vi "System7PressureTemp.vi"() -> ()   [LabVIEW 2015]
uses:
  Control 1.ctl
  <vilib>/DAQmx/write.llb/DAQmx Write (Digital 1D Bool NChan 1Samp 1Line).vi
  <vilib>/DAQmx/write.llb/DAQmx Write (Digital Bool 1Line 1Point).vi
  <vilib>/DAQmx/read.llb/DAQmx Read (Analog DBL 1Chan 1Samp).vi
  <vilib>/DAQmx/read.llb/DAQmx Read (Analog 1D Wfm NChan NSamp).vi
  <vilib>/Analysis/baseanly.llb/Mean (DBL).vi
  <vilib>/DAQmx/write.llb/DAQmx Write (Analog DBL 1Chan 1Samp).vi
  <vilib>/DAQmx/miscellaneous.llb/DAQmx Fill In Error Info.vi
  <vilib>/addons/control/pid/NI_PID_autopid.lvlib
  <vilib>/Analysis/NI_AALBase.lvlib
panel:
  out "Voltage Reading(Temp) 2":dbl format="%#_13g"
  out "Temperature (Celcius) 2":dbl format="%#.1g"
  out "Temp(C) 2":dbl(slide) scale=-10.0..100.0
  out "Temp Chart 3":waveform(dbl)(graph)
  in  "autotuning parameters 4":T1={"controller type"=1, "relay cycles"=3, "relay amplitude"=1.0, "control specification"=2, "PV noise level"=0.1} {"PV noise level" format="%.2f"; "control specification" items=["normal", "fast", "slow"]; "relay amplitude" format="%.2f"; "controller type" items=["PID", "PI", "P"]}
  in  "PID gains 4":T2={"proportional gain (Kc)"=1.0, "integral time (Ti, min)"=0.01, "derivative time (Td, min)"=0.0} {"derivative time (Td, min)" format="%.3f"; "integral time (Ti, min)" format="%.3f"; "proportional gain (Kc)" format="%.3f"}
  out "PID gains out 4":T2={"proportional gain (Kc)"=1.0, "integral time (Ti, min)"=0.01, "derivative time (Td, min)"=0.0} {"derivative time (Td, min)" format="%.3f"; "integral time (Ti, min)" format="%.3f"; "proportional gain (Kc)" format="%.3f"}
  in  "autotune? (F) 4":bool
  in  "reinitialize? (F) 4":bool
  in  "setpoint in C 2":dbl format="%.2f"
  in  "Manual Control 4":bool
  in  "Heater On/Off 2":bool
  out "Voltage Reading(Temp)":dbl format="%#_13g"
  out "Temperature (Celcius)":dbl format="%#.1g"
  out "Temp(C)":dbl(slide) scale=-10.0..100.0
  out "Temp Chart 2":waveform(dbl)(graph)
  in  "autotuning parameters 3":T1={"controller type"=1, "relay cycles"=3, "relay amplitude"=1.0, "control specification"=2, "PV noise level"=0.1} {"PV noise level" format="%.2f"; "control specification" items=["normal", "fast", "slow"]; "relay amplitude" format="%.2f"; "controller type" items=["PID", "PI", "P"]}
  in  "PID gains 3":T2={"proportional gain (Kc)"=1.0, "integral time (Ti, min)"=0.01, "derivative time (Td, min)"=0.0} {"derivative time (Td, min)" format="%.3f"; "integral time (Ti, min)" format="%.3f"; "proportional gain (Kc)" format="%.3f"}
  out "PID gains out 3":T2={"proportional gain (Kc)"=1.0, "integral time (Ti, min)"=0.01, "derivative time (Td, min)"=0.0} {"derivative time (Td, min)" format="%.3f"; "integral time (Ti, min)" format="%.3f"; "proportional gain (Kc)" format="%.3f"}
  in  "autotune? (F) 3":bool
  in  "reinitialize? (F) 3":bool
  in  "setpoint in C":dbl format="%.2f"
  out "Control Value 3":dbl
  in  "Manual Control 3":bool
  in  "Heater On/Off":bool
  in  "Open/Close (Green)":bool
  in  "Open/Close (Blue)":bool
  in  "Stop program":bool
  in  "On/Off":bool
  in  "Manual Control 2":bool
  in  "Voltage setting 2":dbl format="%#_13g"
  out "Voltage Reading(pressure) 2":dbl format="%#_13g"
  out "Pressure 2":dbl format="%#.3g"
  out "Pressure Chart 2":dbl(graph)
  in  "autotuning parameters 2":T1={"controller type"=1, "relay cycles"=3, "relay amplitude"=1.0, "control specification"=2, "PV noise level"=0.1} {"PV noise level" format="%.2f"; "control specification" items=["normal", "fast", "slow"]; "relay amplitude" format="%.2f"; "controller type" items=["PID", "PI", "P"]}
  in  "PID gains 2":T2={"proportional gain (Kc)"=1.0, "integral time (Ti, min)"=0.01, "derivative time (Td, min)"=0.0} {"derivative time (Td, min)" format="%.3f"; "integral time (Ti, min)" format="%.3f"; "proportional gain (Kc)" format="%.3f"}
  out "PID gains out 2":T2={"proportional gain (Kc)"=1.0, "integral time (Ti, min)"=0.01, "derivative time (Td, min)"=0.0} {"derivative time (Td, min)" format="%.3f"; "integral time (Ti, min)" format="%.3f"; "proportional gain (Kc)" format="%.3f"}
  in  "autotune? (F) 2":bool
  in  "reinitialize? (F) 2":bool
  in  "setpoint in Bar 2":dbl format="%#.5f"
  out "Control Value 2":dbl
  in  "Voltage setting":dbl format="%#_13g"
  in  "Manual Control":bool
  out "Control Value":dbl
  in  "setpoint in Bar":dbl format="%#.5f"
  in  "reinitialize? (F)":bool
  in  "autotune? (F)":bool
  out "PID gains out":T2={"proportional gain (Kc)"=1.0, "integral time (Ti, min)"=0.01, "derivative time (Td, min)"=0.0} {"derivative time (Td, min)" format="%.3f"; "integral time (Ti, min)" format="%.3f"; "proportional gain (Kc)" format="%.3f"}
  in  "PID gains":T2={"proportional gain (Kc)"=1.0, "integral time (Ti, min)"=0.01, "derivative time (Td, min)"=0.0} {"derivative time (Td, min)" format="%.3f"; "integral time (Ti, min)" format="%.3f"; "proportional gain (Kc)" format="%.3f"}
  in  "autotuning parameters":T1={"controller type"=1, "relay cycles"=3, "relay amplitude"=1.0, "control specification"=2, "PV noise level"=0.1} {"PV noise level" format="%.2f"; "control specification" items=["normal", "fast", "slow"]; "relay amplitude" format="%.2f"; "controller type" items=["PID", "PI", "P"]}
  out "Pressure Chart":dbl(graph)
  out "Pressure":dbl format="%#.3g"
  out "Voltage Reading(pressure)":dbl format="%#_13g"
  # "Valves"
  # "Pump 3"
  # "Pressure Vessel 2"
  # "Pressure Vessel 1"
  # "Readings"
  # "Controls"
  # "Readings"
  # "Controls"
  # "PID Settings"
  # "51.12139\n\n0.044676"
  # "Temperature 1"
  # "Temperature 2"
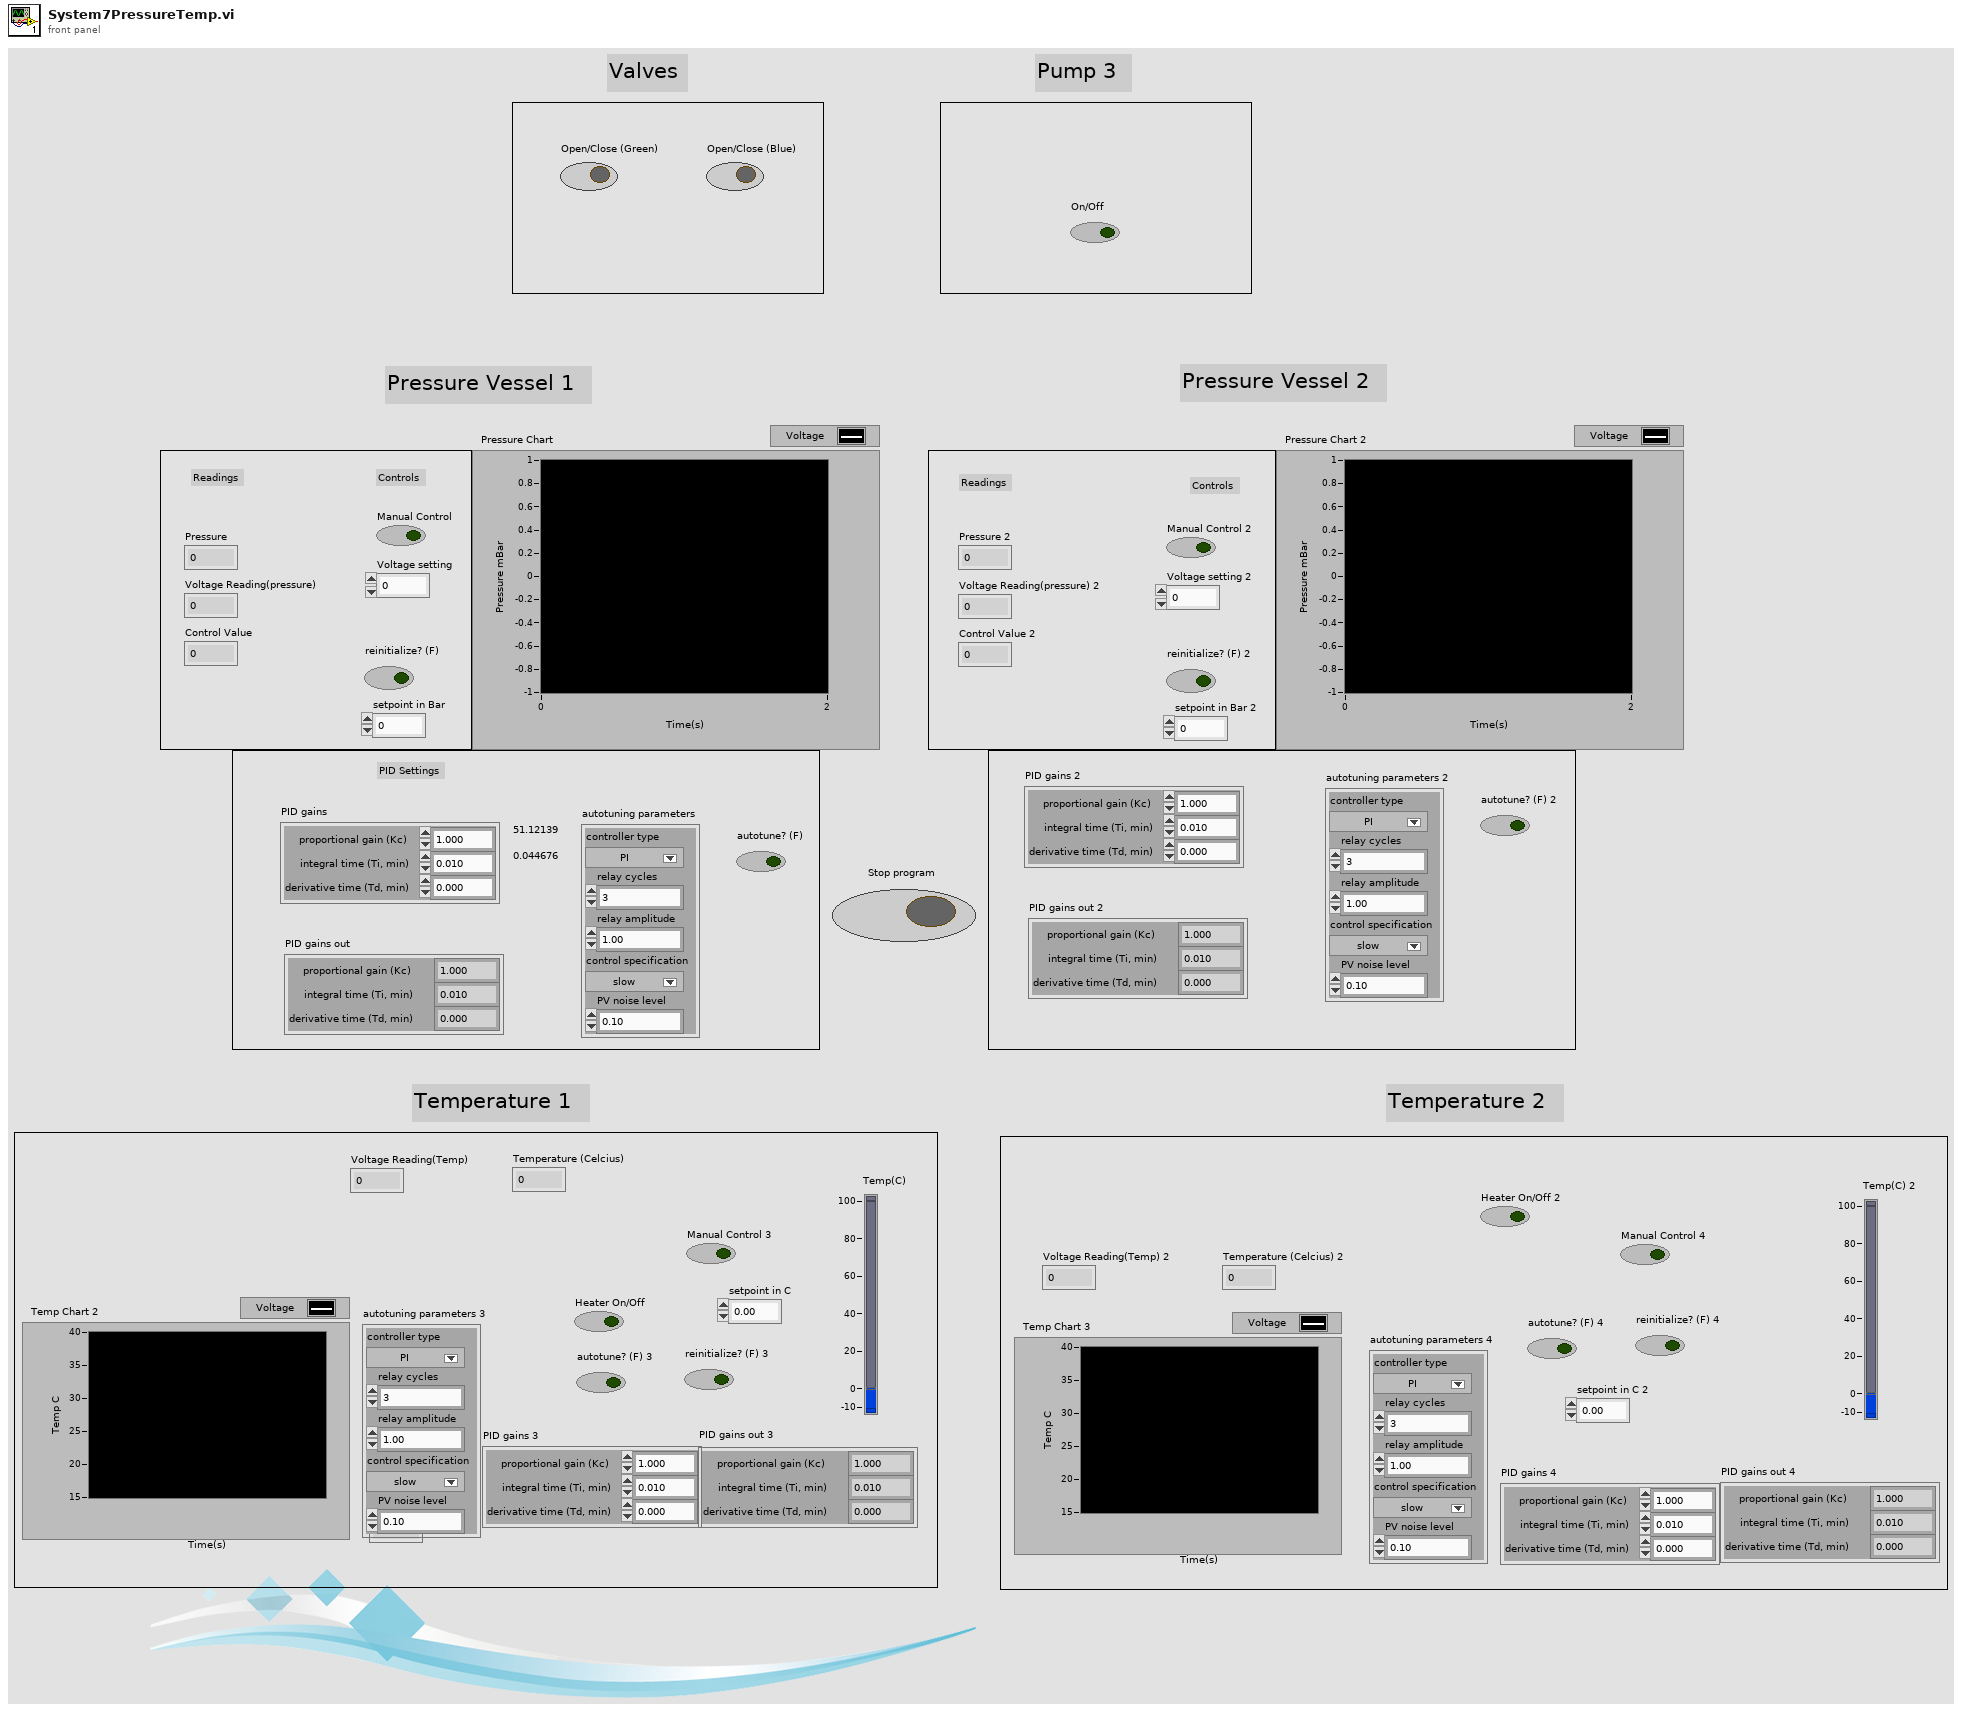
[diagram p1: front panel]
types:
  T1 = cluster{"controller type":u16, "relay cycles":i32, "relay amplitude":dbl, "control specification":u16, "PV noise level":dbl}
  T2 = cluster{"proportional gain (Kc)":dbl, "integral time (Ti, min)":dbl, "derivative time (Td, min)":dbl}
  T3 = typedef "Control 1.ctl" = refnum<k21>
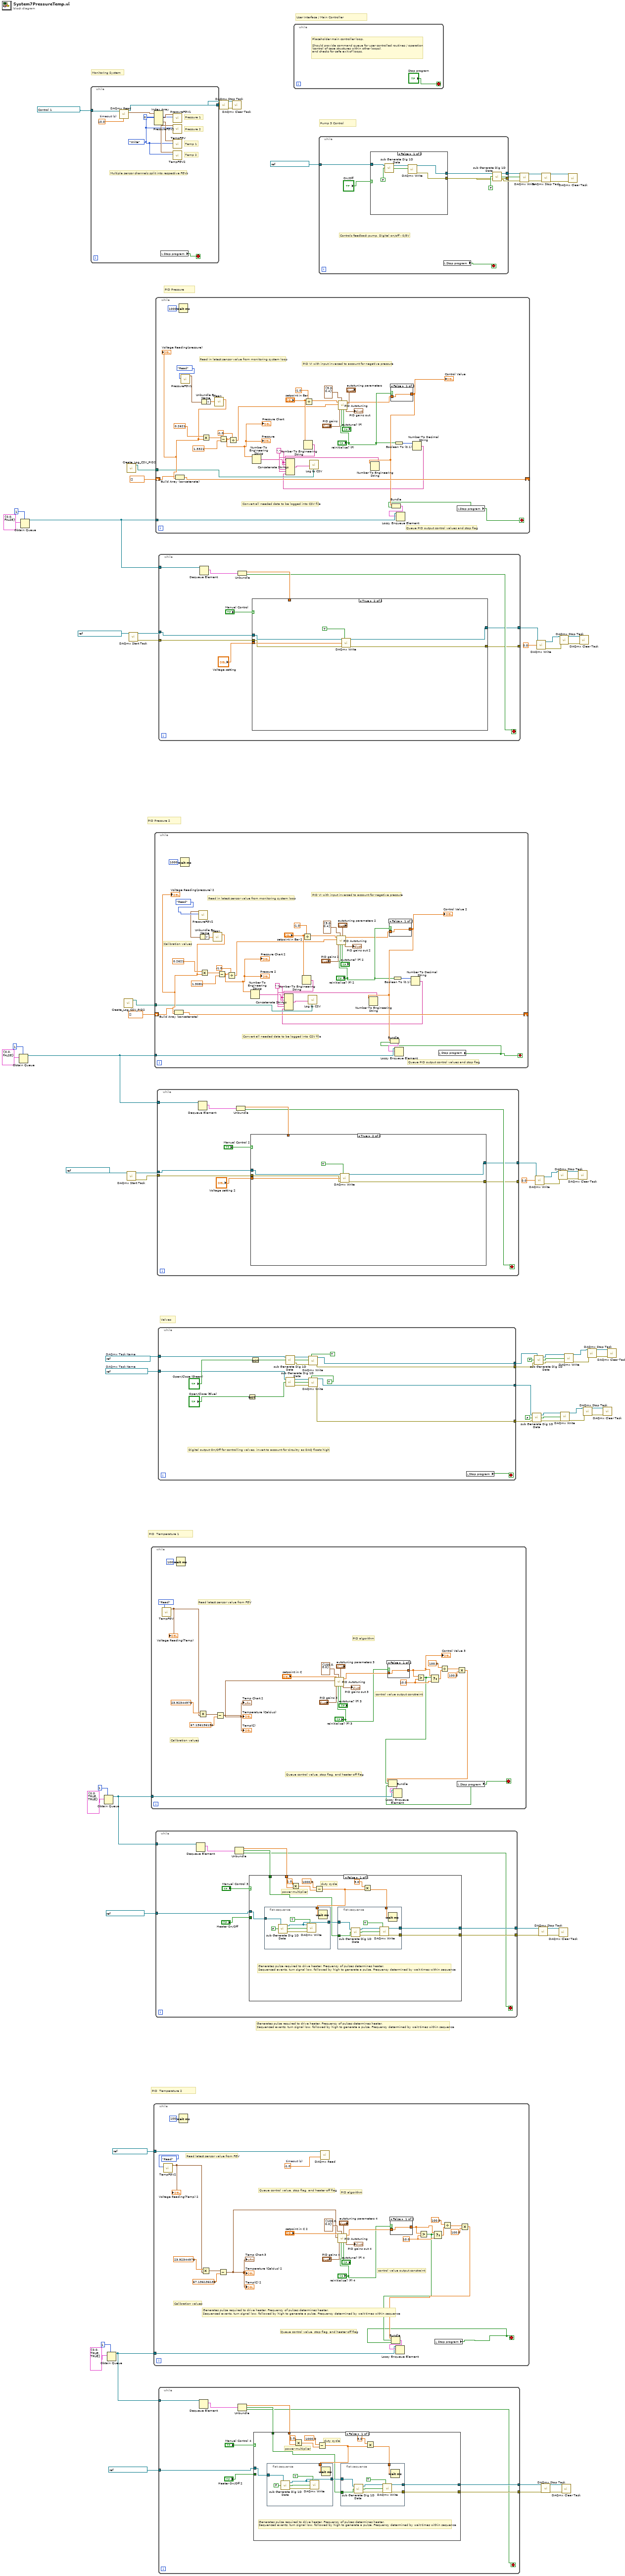
[diagram p0: block diagram]
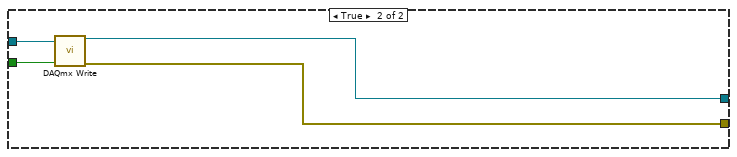
[diagram p2: hidden frame]
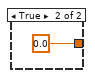
[diagram p3: hidden frame]
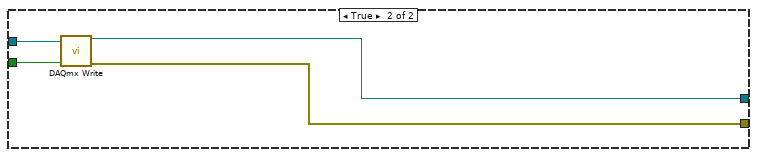
[diagram p4: hidden frame]
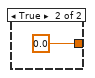
[diagram p5: hidden frame]
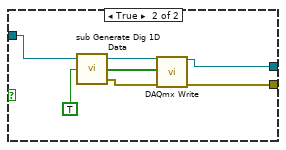
[diagram p6: hidden frame]
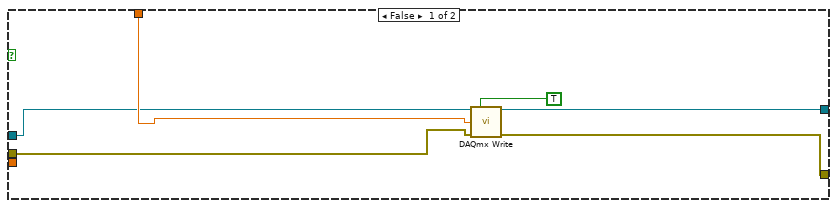
[diagram p7: hidden frame]
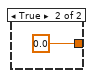
[diagram p8: hidden frame]
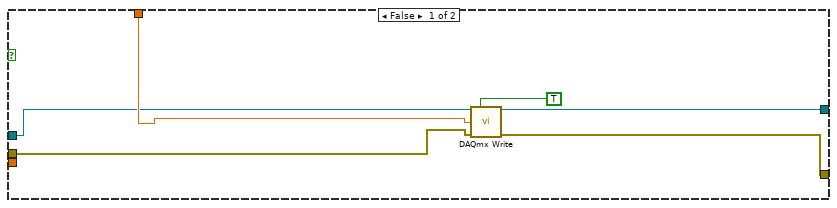
[diagram p9: hidden frame]
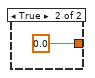
[diagram p10: hidden frame]
diagram:
  w42 = refnum<k21> "NewDigitalSystemBlue"  # DAQmx Task Name
  w43 = refnum<k21> "NewDigitalSystemGreen"  # DAQmx Task Name
  # "Generates pulse required to drive heater. Frequency of pulses determines heater.\nSequenced events, turn signal low, followed by high to generate a pulse. Frequency determined by wait times within sequence"
  # "User Interface / Main Controller"
  # "Pump 3 Control"
  # "PID  Temperature 2"
  # "PID  Temperature 1"
  # "Monitoring System"
  # "Valves"
  # "PID Pressure"
  # "PID Pressure 2"
  n1 = Obtain Queue(max queue size (-1, unlimited)=1, element data type=cluster{dbl, bool} {0.0, FALSE}) -> (queue out=w67:refnum<queue>)  [unwired: 3 in, 2 out]
  n2 = Obtain Queue(max queue size (-1, unlimited)=1, element data type=cluster{dbl, bool} {0.0, FALSE}) -> (queue out=w81:refnum<queue>)  [unwired: 3 in, 2 out]
  n3 = while {
    tunnel: T3 "New AnalogSystemAI0" -> [w91]
    tunnel: [w90] -> w18
    stop <- w93 stop-if-true
    w83 = enum16{"Write", "Read"}."Write" ("Command")
    w92 = 10.0  # timeout (s)
    # "Multiple sensor channels split into respective FGVs"
    # "Temp 2"
    # "Temp 1"
    # "Pressure 2"
    # "Pressure 1"
    n4 = call-poly <vilib>:"DAQmx Read.vi"("task/channels in"=w91, "timeout"=w92) -> ("task out"=w90:refnum<k21>, "data"=w88:waveform(dbl)[])  [unwired: 11 in, 1 out]
    n5 = Index Array(array=w88, index #1=0 ("index")) -> (element #1=w87:waveform(dbl), element #2=w86:waveform(dbl), element #3=w85:waveform(dbl), element #4=w84:waveform(dbl))  [unwired: 3 in]
    n6 = local read "Stop program"() -> (w93:bool)
    n7 = call "PressureFGV1.vi"("Command"=w83, "element"=w87) -> ()  [unwired: 9 in, 1 out]
    n8 = call "PressureFGV2.vi"("Command"=w83, "element"=w86) -> ()  [unwired: 9 in, 1 out]
    n9 = call "TempFGV.vi"("Command"=w83, "element 3"=w85) -> ()  [unwired: 9 in, 1 out]
    n10 = call "TempFGV2.vi"("Command"=w83, "element 3"=w84) -> ()  [unwired: 9 in, 1 out]
  }
  n11 = Obtain Queue(max queue size (-1, unlimited)=1, element data type=cluster{dbl, bool, bool} {0.0, TRUE, TRUE}) -> (queue out=w11:refnum<queue>)  [unwired: 3 in, 2 out]
  n12 = Obtain Queue(max queue size (-1, unlimited)=1, element data type=cluster{dbl, bool, bool} {0.0, TRUE, TRUE}) -> (queue out=w7:refnum<queue>)  [unwired: 3 in, 2 out]
  n13 = call "Create_Log_CSV_PID2.vi"() -> ("path"=w63:path)  [unwired: 11 in]
  n14 = call "Create_Log_CSV_PID2.vi"() -> ("path"=w77:path)  [unwired: 11 in]
  n15 = call <vilib>:"DAQmx Start Task.vi"("task/channels in"=refnum<k21> "NewAnalogSystemAO1") -> ("task out"=w62:refnum<k21>, "error out"=w61:errorcluster)  [unwired: 13 in]
  n16 = call <vilib>:"DAQmx Start Task.vi"("task/channels in"=refnum<k21> "NewAnalogSystemAO0") -> ("task out"=w76:refnum<k21>, "error out"=w75:errorcluster)  [unwired: 13 in]
  n17 = while {
    tunnel: w11 -> [w97]
    stop <- w96 stop-if-true
    w103 = 10.0 ("f")
    # "Queue control value, stop flag, and heater off flag"
    # "Calibration values"
    # "control value output constraint"
    # "PID algorithm"
    # "Read latest sensor value from FGV"
    n18 = call "TempFGV.vi"("Command"=enum16{"Write", "Read"}."Read") -> ("element 2"=w94:waveform(dbl))  [unwired: 10 in]
    "Voltage Reading(Temp)" <- w94
    n19 = Wait (ms)(milliseconds to wait=u32 100) -> ()  [unwired: 1 out]
    n20 = Multiply(x=23.92344976, y=w94) -> (x*y=w118:waveform(dbl))
    n21 = Subtract(x=w118, y=67.136136136) -> (x-y=w101:waveform(dbl))
    "Temperature (Celcius)" <- w101
    "Temp(C)" <- w101
    "Temp Chart 2" <- w101
    n22 = call <vilib>:"PID Autotuning.vi"("autotune? (F)"="autotune? (F) 3", "autotuning parameters"="autotuning parameters 3", "reinitialize? (F)"="reinitialize? (F) 3", "output range"=cluster{"output high":dbl, "output low":dbl} {"output high"=100.0, "output low"=0.0}, "PID gains"="PID gains 3", "process variable"=w101, "setpoint"="setpoint in C") -> ("PID gains out"=→"PID gains out 3":T2, "output"=w111:dbl)  [unwired: 1 in, 2 out]
    n23 = case shown="False" "reinitialize? (F) 3" {
      tunnel: [w120 0.0] -> w104
      tunnel: w111 -> [w120 _]
      frame False {
      }
      frame True {
      }
    }
    "Control Value 3" <- w104
    n24 = Greater?(x=w104, y=w103) -> (0:w99:bool)
    n25 = Select(t=w104, s=w99, f=w103) -> (s? t:f=w105:dbl)
    n26 = Divide(x=100.0, y=w105) -> (x/y=w107:dbl)
    n27 = local read "Stop program"() -> (w96:bool)
    n28 = Multiply(x=w107, y=100.0) -> (x*y=w100:dbl)
    n29 = Bundle(w100, w99, "Stop program"=w96) -> (w98:cluster{dbl, bool, "Stop program":bool})  [unwired: 1 in]
    n30 = Lossy Enqueue Element(queue=w97, element=w98) -> ()  [unwired: 1 in, 4 out]
  }
  n31 = while {
    tunnel: refnum<k21> "MyVoltageTask_0" -> [w145]
    tunnel: w7 -> [w125]
    stop <- w122 stop-if-true
    w131 = 10.0 ("f")
    w149 = -1.0  # timeout (s)
    # "Generates pulse required to drive heater. Frequency of pulses determines heater.\nSequenced events, turn signal low, followed by high to generate a pulse. Frequency determined by wait times within sequence"
    # "Queue control value, stop flag, and heater off flag"
    # "Queue control value, stop flag, and heater off flag"
    # "Calibration values"
    # "control value output constraint"
    # "PID algorithm"
    # "Read latest sensor value from FGV"
    n32 = call "TempFGV2.vi"("Command"=enum16{"Write", "Read"}."Read") -> ("element 2"=w123:waveform(dbl))  [unwired: 10 in]
    "Voltage Reading(Temp) 2" <- w123
    n33 = Wait (ms)(milliseconds to wait=u32 100) -> ()  [unwired: 1 out]
    n34 = Multiply(x=23.92344976, y=w123) -> (x*y=w147:waveform(dbl))
    n35 = Subtract(x=w147, y=67.136136136) -> (x-y=w129:waveform(dbl))
    "Temperature (Celcius) 2" <- w129
    "Temp(C) 2" <- w129
    "Temp Chart 3" <- w129
    n36 = call-poly <vilib>:"DAQmx Read.vi"("task/channels in"=w145, "timeout"=w149) -> ()  [unwired: 11 in, 3 out]
    n37 = call <vilib>:"PID Autotuning.vi"("autotune? (F)"="autotune? (F) 4", "autotuning parameters"="autotuning parameters 4", "reinitialize? (F)"="reinitialize? (F) 4", "output range"=cluster{"output high":dbl, "output low":dbl} {"output high"=100.0, "output low"=0.0}, "PID gains"="PID gains 4", "process variable"=w129, "setpoint"="setpoint in C 2") -> ("PID gains out"=→"PID gains out 4":T2, "output"=w139:dbl)  [unwired: 1 in, 2 out]
    n38 = case shown="False" "reinitialize? (F) 4" {
      tunnel: [w150 0.0] -> w132
      tunnel: w139 -> [w150 _]
      frame False {
      }
      frame True {
      }
    }
    n39 = Greater?(x=w132, y=w131) -> (0:w127:bool)
    n40 = Select(t=w132, s=w127, f=w131) -> (s? t:f=w133:dbl)
    n41 = local read "Stop program"() -> (w122:bool)
    n42 = Divide(x=100.0, y=w133) -> (x/y=w135:dbl)
    n43 = Multiply(x=w135, y=100.0) -> (x*y=w128:dbl)
    n44 = Bundle(w128, w127, "Stop program"=w122) -> (w126:cluster{dbl, bool, "Stop program":bool})  [unwired: 1 in]
    n45 = Lossy Enqueue Element(queue=w125, element=w126) -> ()  [unwired: 1 in, 4 out]
  }
  n46 = while {
    tunnel: w67 -> [w178]
    shift-right: [w175] -> _
    shift-left: dbl[] [] -> [w176]
    tunnel: w63 -> [w169]
    stop <- w156 stop-if-true
    w164 = ","
    # "Calibration values"
    # "Queue PID output control values and stop flag"
    # "Convert all needed data to be logged into CSV file"
    # "PID VI with input inversed to account for negative pressure"
    # "Read in latest sensor value from monitoring system loop"
    n47 = Wait (ms)(milliseconds to wait=u32 1000) -> ()  [unwired: 1 out]
    n48 = call "PressureFGV2.vi"("Command"=enum16{"Write", "Read"}."Read") -> ("element 2"=w152:waveform(dbl))  [unwired: 10 in]
    n49 = Unbundle By Name(w152) -> ("Y"=w154:dbl[])
    n50 = call-poly <vilib>:"Mean.vi"("X"=w154) -> ("mean"=w177:dbl)  [unwired: 1 out]
    "Voltage Reading(pressure) 2" <- w177
    n51 = Build Array (concatenate)(w176, w177) -> (w175:dbl[])
    n52 = Multiply(x=0.2621, y=w177) -> (x*y=w185:dbl)
    n53 = Subtract(x=w185, y=1.3081) -> (x-y=w173:dbl)
    "Pressure 2" <- w173
    "Pressure Chart 2" <- w173
    n54 = Divide(x=w173, y=-1.0) -> (x/y=w161:dbl)
    n55 = Number To Engineering String(4:w173) -> (0:w168:string)  [unwired: 3 in]
    n56 = Number To Engineering String(4:"setpoint in Bar 2") -> (0:w167:string)  [unwired: 3 in]
    n57 = Divide(x="setpoint in Bar 2", y=-1.0) -> (x/y=w160:dbl)
    n58 = call <vilib>:"PID Autotuning.vi"("autotune? (F)"="autotune? (F) 2", "autotuning parameters"="autotuning parameters 2", "reinitialize? (F)"="reinitialize? (F) 2", "output range"=cluster{"output high":dbl, "output low":dbl} {"output high"=5.0, "output low"=0.4}, "PID gains"="PID gains 2", "process variable"=w161, "setpoint"=w160) -> ("PID gains out"=→"PID gains out 2":T2, "output"=w158:dbl)  [unwired: 1 in, 2 out]
    n59 = case shown="False" "reinitialize? (F) 2" {
      tunnel: [w187 0.0] -> w172
      tunnel: w158 -> [w187 _]
      frame False {
      }
      frame True {
      }
    }
    "Control Value 2" <- w172
    n60 = Number To Engineering String(4:w172) -> (0:w171:string)  [unwired: 3 in]
    n61 = Boolean To (0,1)(Boolean="reinitialize? (F) 2") -> (0, 1=w165:i16)
    n62 = Number To Decimal String(number=w165) -> (decimal integer string=w163:string)  [unwired: 1 in]
    n63 = Concatenate Strings(w167, w164, w168, w164, w171, w164, w163) -> (w170:string)
    n64 = call "Log to CSV.vi"("Data Str"=w170, "Path"=w169) -> ()  [unwired: 5 in, 1 out]
    n65 = local read "Stop program"() -> (w156:bool)
    n66 = Bundle("output"=w172, "Stop program"=w156) -> (w157:cluster{"output":dbl, "Stop program":bool})  [unwired: 1 in]
    n67 = Lossy Enqueue Element(queue=w178, element=w157) -> ()  [unwired: 1 in, 4 out]
  }
  n68 = while {
    tunnel: w11 -> [w198]
    tunnel: refnum<k21> "MyDigitalOutTask_2" -> [w195]
    tunnel: [w191] -> w14
    tunnel: [w190] -> w15
    stop <- w189 stop-if-true
    n69 = Dequeue Element(queue=w198) -> (element=w194:cluster{dbl, bool, bool})  [unwired: 2 in, 3 out]
    n70 = Unbundle(w194) -> (w193:dbl, w192:bool, w189:bool)
    n71 = case shown="False" "Manual Control 3" {
      tunnel: w195 -> [w209 w230]
      tunnel: "Heater On/Off" -> [_ w229]
      tunnel: w193 -> [w208 _]
      tunnel: w192 -> [w203 _]
      tunnel: [w200 w228] -> w191
      tunnel: [w199 w227] -> w190
      frame False {
        # "Generates pulse required to drive heater. Frequency of pulses determines heater.\nSequenced events, turn signal low, followed by high to generate a pulse. Frequency determined by wait times within sequence"
        # "duty cycle"
        # "power multiplier"
        n72 = flat-sequence {
          tunnel: w209 -> [w223]
          tunnel: [w222] -> w210
          tunnel: w207 -> [w221]
          frame #0 {
            n73 = call <vilib>:"sub Generate Dig 1D Data.vi"("initial value"=FALSE, "task in"=w223) -> ("error out"=w225:errorcluster, "Data"=w226:bool[], "task out"=w222:refnum<k21>)  [unwired: 1 in]
            n74 = call-poly <vilib>:"DAQmx Write.vi"("task/channels in"=w222, "auto start"=TRUE, "data"=w226, "error in"=w225) -> ()  [unwired: 9 in, 3 out]
            n75 = Wait (ms)(milliseconds to wait=w221) -> ()  [unwired: 1 out]
          }
        }
        n76 = Multiply(x=1.0, y=w208) -> (x*y=w202:dbl)
        n77 = Subtract(x=1000.0, y=w202) -> (x-y=w207:dbl)
        n78 = flat-sequence {
          tunnel: w210 -> [w215]
          tunnel: w205 -> [w214]
          tunnel: w203 -> [w213]
          tunnel: [w212] -> w200
          tunnel: [w211] -> w199
          frame #0 {
            n79 = call <vilib>:"sub Generate Dig 1D Data.vi"("initial value"=w213, "task in"=w215) -> ("error out"=w218:errorcluster, "Data"=w216:bool[], "task out"=w217:refnum<k21>)  [unwired: 1 in]
            n80 = call-poly <vilib>:"DAQmx Write.vi"("task/channels in"=w217, "auto start"=TRUE, "data"=w216, "error in"=w218) -> ("task out"=w212:refnum<k21>, "error out"=w211:errorcluster)  [unwired: 9 in, 1 out]
            n81 = Wait (ms)(milliseconds to wait=w214) -> ()  [unwired: 1 out]
          }
        }
        n82 = Multiply(x=9.0, y=w207) -> (x*y=w205:dbl)
      }
      frame True {
        n83 = call-poly <vilib>:"DAQmx Write.vi"("task/channels in"=w230, "data"=w229) -> ("task out"=w228:refnum<k21>, "error out"=w227:errorcluster)  [unwired: 11 in, 1 out]
      }
    }
  }
  n84 = while {
    tunnel: w81 -> [w257]
    shift-right: [w252] -> _
    shift-left: dbl[] [] -> [w253]
    tunnel: w77 -> [w246]
    stop <- w234 stop-if-true
    w241 = ","
    # "Queue PID output control values and stop flag"
    # "Convert all needed data to be logged into CSV file"
    # "PID VI with input inversed to account for negative pressure"
    # "Read in latest sensor value from monitoring system loop"
    n85 = Wait (ms)(milliseconds to wait=u32 1000) -> ()  [unwired: 1 out]
    n86 = call "PressureFGV1.vi"("Command"=enum16{"Write", "Read"}."Read") -> ("element 2"=w231:waveform(dbl))  [unwired: 10 in]
    n87 = Unbundle By Name(w231) -> ("Y"=w255:dbl[])
    n88 = call-poly <vilib>:"Mean.vi"("X"=w255) -> ("mean"=w254:dbl)  [unwired: 1 out]
    "Voltage Reading(pressure)" <- w254
    n89 = Build Array (concatenate)(w253, w254) -> (w252:dbl[])
    n90 = Multiply(x=0.2621, y=w254) -> (x*y=w264:dbl)
    n91 = Subtract(x=w264, y=1.3321) -> (x-y=w250:dbl)
    "Pressure" <- w250
    "Pressure Chart" <- w250
    n92 = Divide(x=w250, y=-1.0) -> (x/y=w238:dbl)
    n93 = Number To Engineering String(4:w250) -> (0:w245:string)  [unwired: 3 in]
    n94 = Number To Engineering String(4:"setpoint in Bar") -> (0:w244:string)  [unwired: 3 in]
    n95 = Divide(x="setpoint in Bar", y=-1.0) -> (x/y=w237:dbl)
    n96 = call <vilib>:"PID Autotuning.vi"("autotune? (F)"="autotune? (F)", "autotuning parameters"="autotuning parameters", "reinitialize? (F)"="reinitialize? (F)", "output range"=cluster{"output high":dbl, "output low":dbl} {"output high"=5.0, "output low"=0.4}, "PID gains"="PID gains", "process variable"=w238, "setpoint"=w237) -> ("PID gains out"=→"PID gains out":T2, "output"=w235:dbl)  [unwired: 1 in, 2 out]
    n97 = case shown="False" "reinitialize? (F)" {
      tunnel: [w266 0.0] -> w249
      tunnel: w235 -> [w266 _]
      frame False {
      }
      frame True {
      }
    }
    "Control Value" <- w249
    n98 = Number To Engineering String(4:w249) -> (0:w248:string)  [unwired: 3 in]
    n99 = Boolean To (0,1)(Boolean="reinitialize? (F)") -> (0, 1=w242:i16)
    n100 = Number To Decimal String(number=w242) -> (decimal integer string=w240:string)  [unwired: 1 in]
    n101 = Concatenate Strings(w244, w241, w245, w241, w248, w241, w240) -> (w247:string)
    n102 = call "Log to CSV.vi"("Data Str"=w247, "Path"=w246) -> ()  [unwired: 5 in, 1 out]
    n103 = local read "Stop program"() -> (w234:bool)
    n104 = Bundle("output"=w249, "Stop program"=w234) -> (w256:cluster{"output":dbl, "Stop program":bool})  [unwired: 1 in]
    n105 = Lossy Enqueue Element(queue=w257, element=w256) -> ()  [unwired: 1 in, 4 out]
  }
  n106 = while {
    tunnel: w67 -> [w277]
    tunnel: w62 -> [w275]
    tunnel: [w270] -> w59
    tunnel: w61 -> [w269]
    tunnel: [w268] -> _
    stop <- w271 stop-if-true
    n107 = Dequeue Element(queue=w277) -> (element=w274:cluster{dbl, bool})  [unwired: 2 in, 3 out]
    n108 = Unbundle(w274) -> (w273:dbl, w271:bool)
    n109 = case shown="True" "Manual Control 2" {
      tunnel: w275 -> [w281 w288]
      tunnel: w273 -> [w282 _]
      tunnel: "Voltage setting 2" -> [_ w287]
      tunnel: [w280 w286] -> w270
      tunnel: w269 -> [w279 w285]
      tunnel: [w278 w284] -> w268
      frame False {
        n110 = call-poly <vilib>:"DAQmx Write.vi"("task/channels in"=w281, "auto start"=TRUE, "data"=w282, "error in"=w279) -> ("task out"=w280:refnum<k21>, "error out"=w278:errorcluster)  [unwired: 9 in, 1 out]
      }
      frame True {
        n111 = call-poly <vilib>:"DAQmx Write.vi"("task/channels in"=w288, "auto start"=TRUE, "data"=w287, "error in"=w285) -> ("task out"=w286:refnum<k21>, "error out"=w284:errorcluster)  [unwired: 9 in, 1 out]
      }
    }
  }
  n112 = while {
    tunnel: w43 -> [w298]
    tunnel: w42 -> [w297]
    tunnel: [w296] -> w32
    tunnel: [w295] -> w28
    tunnel: [w292] -> w25
    tunnel: [w291] -> w23
    stop <- w290 stop-if-true
    # "Digital output On/Off for controlling valves, invert to account for circuitry as DAQ floats high"
    n113 = Not(x="Open/Close (Blue)") -> (.not. x?=w308:bool)
    n114 = Not(x="Open/Close (Green)") -> (.not. x?=w307:bool)
    n115 = call <vilib>:"sub Generate Dig 1D Data.vi"("initial value"=w307, "task in"=w298) -> ("error out"=w294:errorcluster, "Data"=w305:bool[], "task out"=w302:refnum<k21>)  [unwired: 1 in]
    n116 = call <vilib>:"sub Generate Dig 1D Data.vi"("initial value"=w308, "task in"=w297) -> ("error out"=w293:errorcluster, "Data"=w304:bool[], "task out"=w303:refnum<k21>)  [unwired: 1 in]
    n117 = call-poly <vilib>:"DAQmx Write.vi"("task/channels in"=w302, "auto start"=TRUE, "data"=w305, "error in"=w294) -> ("task out"=w296:refnum<k21>, "error out"=w292:errorcluster)  [unwired: 9 in, 1 out]
    n118 = call-poly <vilib>:"DAQmx Write.vi"("task/channels in"=w303, "auto start"=TRUE, "data"=w304, "error in"=w293) -> ("task out"=w295:refnum<k21>, "error out"=w291:errorcluster)  [unwired: 9 in, 1 out]
    n119 = local read "Stop program"() -> (w290:bool)
  }
  n120 = while {
    tunnel: w7 -> [w318]
    tunnel: refnum<k21> "MyDigitalOutTask_2" -> [w315]
    tunnel: [w311] -> w4
    tunnel: [w310] -> w3
    stop <- w309 stop-if-true
    n121 = Dequeue Element(queue=w318) -> (element=w314:cluster{dbl, bool, bool})  [unwired: 2 in, 3 out]
    n122 = Unbundle(w314) -> (w313:dbl, w312:bool, w309:bool)
    n123 = case shown="False" "Manual Control 4" {
      tunnel: w315 -> [w329 w350]
      tunnel: "Heater On/Off 2" -> [_ w349]
      tunnel: w313 -> [w328 _]
      tunnel: w312 -> [w323 _]
      tunnel: [w320 w348] -> w311
      tunnel: [w319 w347] -> w310
      frame False {
        # "Generates pulse required to drive heater. Frequency of pulses determines heater.\nSequenced events, turn signal low, followed by high to generate a pulse. Frequency determined by wait times within sequence"
        # "duty cycle"
        # "power multiplier"
        n124 = flat-sequence {
          tunnel: w329 -> [w343]
          tunnel: [w342] -> w330
          tunnel: w327 -> [w341]
          frame #0 {
            n125 = call <vilib>:"sub Generate Dig 1D Data.vi"("initial value"=FALSE, "task in"=w343) -> ("error out"=w345:errorcluster, "Data"=w346:bool[], "task out"=w342:refnum<k21>)  [unwired: 1 in]
            n126 = call-poly <vilib>:"DAQmx Write.vi"("task/channels in"=w342, "auto start"=TRUE, "data"=w346, "error in"=w345) -> ()  [unwired: 9 in, 3 out]
            n127 = Wait (ms)(milliseconds to wait=w341) -> ()  [unwired: 1 out]
          }
        }
        n128 = Multiply(x=1.0, y=w328) -> (x*y=w322:dbl)
        n129 = Subtract(x=1000.0, y=w322) -> (x-y=w327:dbl)
        n130 = flat-sequence {
          tunnel: w330 -> [w335]
          tunnel: w325 -> [w334]
          tunnel: w323 -> [w333]
          tunnel: [w332] -> w320
          tunnel: [w331] -> w319
          frame #0 {
            n131 = call <vilib>:"sub Generate Dig 1D Data.vi"("initial value"=w333, "task in"=w335) -> ("error out"=w338:errorcluster, "Data"=w336:bool[], "task out"=w337:refnum<k21>)  [unwired: 1 in]
            n132 = call-poly <vilib>:"DAQmx Write.vi"("task/channels in"=w337, "auto start"=TRUE, "data"=w336, "error in"=w338) -> ("task out"=w332:refnum<k21>, "error out"=w331:errorcluster)  [unwired: 9 in, 1 out]
            n133 = Wait (ms)(milliseconds to wait=w334) -> ()  [unwired: 1 out]
          }
        }
        n134 = Multiply(x=9.0, y=w327) -> (x*y=w325:dbl)
      }
      frame True {
        n135 = call-poly <vilib>:"DAQmx Write.vi"("task/channels in"=w350, "data"=w349) -> ("task out"=w348:refnum<k21>, "error out"=w347:errorcluster)  [unwired: 11 in, 1 out]
      }
    }
  }
  n136 = while {
    tunnel: w81 -> [w360]
    tunnel: w76 -> [w358]
    tunnel: [w353] -> w73
    tunnel: w75 -> [w352]
    tunnel: [w351] -> _
    stop <- w354 stop-if-true
    n137 = Dequeue Element(queue=w360) -> (element=w357:cluster{dbl, bool})  [unwired: 2 in, 3 out]
    n138 = Unbundle(w357) -> (w356:dbl, w354:bool)
    n139 = case shown="True" "Manual Control" {
      tunnel: w358 -> [w364 w371]
      tunnel: w356 -> [w365 _]
      tunnel: "Voltage setting" -> [_ w370]
      tunnel: [w363 w369] -> w353
      tunnel: w352 -> [w362 w368]
      tunnel: [w361 w367] -> w351
      frame False {
        n140 = call-poly <vilib>:"DAQmx Write.vi"("task/channels in"=w364, "auto start"=TRUE, "data"=w365, "error in"=w362) -> ("task out"=w363:refnum<k21>, "error out"=w361:errorcluster)  [unwired: 9 in, 1 out]
      }
      frame True {
        n141 = call-poly <vilib>:"DAQmx Write.vi"("task/channels in"=w371, "auto start"=TRUE, "data"=w370, "error in"=w368) -> ("task out"=w369:refnum<k21>, "error out"=w367:errorcluster)  [unwired: 9 in, 1 out]
      }
    }
  }
  n142 = call <vilib>:"DAQmx Stop Task.vi"("task/channels in"=w18) -> ("task out"=w20:refnum<k21>, "error out"=w19:errorcluster)  [unwired: 13 in]
  n143 = call <vilib>:"DAQmx Clear Task.vi"("task in"=w20, "error in"=w19) -> ()  [unwired: 13 in, 1 out]
  n144 = while {
    stop <- "Stop program" stop-if-true
    # "Placeholder main controller loop.\n\nShould provide command queue for user controlled routines / operation \n(control of case structures within other loops), \nand checks for safe exit of loops."
  }
  n145 = while {
    tunnel: refnum<k21> "NewDigSystemP0L2" -> [w377]
    tunnel: [w376] -> w47
    tunnel: [w375] -> w46
    stop <- w374 stop-if-true
    # "Controls feedback pump, Digital on/off - 0/5V"
    n146 = case shown="False" "On/Off" {
      tunnel: w377 -> [w384 w388]
      tunnel: [w380 w387] -> w376
      tunnel: [w379 w385] -> w375
      frame False {
        n147 = call <vilib>:"sub Generate Dig 1D Data.vi"("initial value"=FALSE, "task in"=w384) -> ("Data"=w382:bool[], "task out"=w383:refnum<k21>)  [unwired: 1 in, 1 out]
        n148 = call-poly <vilib>:"DAQmx Write.vi"("task/channels in"=w383, "data"=w382) -> ("task out"=w380:refnum<k21>, "error out"=w379:errorcluster)  [unwired: 11 in, 1 out]
      }
      frame True {
        n149 = call <vilib>:"sub Generate Dig 1D Data.vi"("initial value"=TRUE, "task in"=w388) -> ("error out"=w386:errorcluster, "Data"=w390:bool[], "task out"=w389:refnum<k21>)  [unwired: 1 in]
        n150 = call-poly <vilib>:"DAQmx Write.vi"("task/channels in"=w389, "data"=w390, "error in"=w386) -> ("task out"=w387:refnum<k21>, "error out"=w385:errorcluster)  [unwired: 10 in, 1 out]
      }
    }
    n151 = local read "Stop program"() -> (w374:bool)
  }
  n152 = call <vilib>:"sub Generate Dig 1D Data.vi"("error in"=w46, "initial value"=FALSE, "task in"=w47) -> ("error out"=w51:errorcluster, "Data"=w49:bool[], "task out"=w50:refnum<k21>)
  n153 = call-poly <vilib>:"DAQmx Write.vi"("task/channels in"=w50, "data"=w49, "error in"=w51) -> ("task out"=w45:refnum<k21>, "error out"=w44:errorcluster)  [unwired: 10 in, 1 out]
  n154 = call <vilib>:"sub Generate Dig 1D Data.vi"("error in"=w23, "initial value"=FALSE, "task in"=w28) -> ("error out"=w22:errorcluster, "Data"=w27:bool[], "task out"=w29:refnum<k21>)
  n155 = call <vilib>:"sub Generate Dig 1D Data.vi"("error in"=w25, "initial value"=FALSE, "task in"=w32) -> ("error out"=w24:errorcluster, "Data"=w26:bool[], "task out"=w33:refnum<k21>)
  n156 = call-poly <vilib>:"DAQmx Write.vi"("task/channels in"=w59, "data"=0.0) -> ("task out"=w58:refnum<k21>, "error out"=w57:errorcluster)  [unwired: 11 in, 1 out]
  n157 = call-poly <vilib>:"DAQmx Write.vi"("task/channels in"=w73, "data"=0.0) -> ("task out"=w72:refnum<k21>, "error out"=w71:errorcluster)  [unwired: 11 in, 1 out]
  n158 = call <vilib>:"DAQmx Stop Task.vi"("task/channels in"=w14, "error in"=w15) -> ("task out"=w16:refnum<k21>, "error out"=w17:errorcluster)  [unwired: 12 in]
  n159 = call <vilib>:"DAQmx Stop Task.vi"("task/channels in"=w4, "error in"=w3) -> ("task out"=w2:refnum<k21>, "error out"=w1:errorcluster)  [unwired: 12 in]
  n160 = call <vilib>:"DAQmx Stop Task.vi"("task/channels in"=w45, "error in"=w44) -> ("task out"=w53:refnum<k21>, "error out"=w52:errorcluster)  [unwired: 12 in]
  n161 = call <vilib>:"DAQmx Stop Task.vi"("task/channels in"=w58, "error in"=w57) -> ("task out"=w60:refnum<k21>, "error out"=w56:errorcluster)  [unwired: 12 in]
  n162 = call <vilib>:"DAQmx Clear Task.vi"("task in"=w16, "error in"=w17) -> ()  [unwired: 13 in, 1 out]
  n163 = call <vilib>:"DAQmx Stop Task.vi"("task/channels in"=w72, "error in"=w71) -> ("task out"=w74:refnum<k21>, "error out"=w70:errorcluster)  [unwired: 12 in]
  n164 = call-poly <vilib>:"DAQmx Write.vi"("task/channels in"=w29, "data"=w27, "error in"=w22) -> ("task out"=w36:refnum<k21>, "error out"=w35:errorcluster)  [unwired: 10 in, 1 out]
  n165 = call <vilib>:"DAQmx Clear Task.vi"("task in"=w2, "error in"=w1) -> ()  [unwired: 13 in, 1 out]
  n166 = call-poly <vilib>:"DAQmx Write.vi"("task/channels in"=w33, "data"=w26, "error in"=w24) -> ("task out"=w39:refnum<k21>, "error out"=w40:errorcluster)  [unwired: 10 in, 1 out]
  n167 = call <vilib>:"DAQmx Clear Task.vi"("task in"=w53, "error in"=w52) -> ()  [unwired: 13 in, 1 out]
  n168 = call <vilib>:"DAQmx Clear Task.vi"("task in"=w60, "error in"=w56) -> ()  [unwired: 13 in, 1 out]
  n169 = call <vilib>:"DAQmx Clear Task.vi"("task in"=w74, "error in"=w70) -> ()  [unwired: 13 in, 1 out]
  n170 = call <vilib>:"DAQmx Stop Task.vi"("task/channels in"=w36, "error in"=w35) -> ("task out"=w37:refnum<k21>, "error out"=w34:errorcluster)  [unwired: 12 in]
  n171 = call <vilib>:"DAQmx Stop Task.vi"("task/channels in"=w39, "error in"=w40) -> ("task out"=w38:refnum<k21>, "error out"=w41:errorcluster)  [unwired: 12 in]
  n172 = call <vilib>:"DAQmx Clear Task.vi"("task in"=w37, "error in"=w34) -> ()  [unwired: 13 in, 1 out]
  n173 = call <vilib>:"DAQmx Clear Task.vi"("task in"=w38, "error in"=w41) -> ()  [unwired: 13 in, 1 out]
